vi "NISE.Reserve.vi"(0 "SLSC Interface in":refnum<class "SLSC Interface.lvclass">, 5 "devices":refnum<k21>="$DefaultDevices", 7 "reservation access (Read/Write)":i32(ring)=3 items=["Read Only"=1, "Read/Write"=3], 9 "reservation group":string, 11 "error in (no error)":errorcluster) -> (4 "SLSC Interface out":refnum<class "SLSC Interface.lvclass">, 15 "error out":errorcluster)   [LabVIEW 2016, in "SLSC Interface.lvclass"]
uses:
  SLSC Interface.lvclass
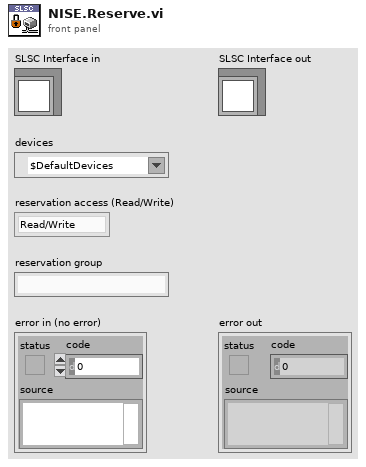
[diagram p1: front panel]
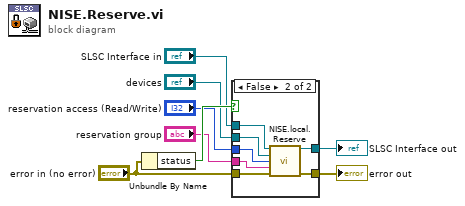
[diagram p0: block diagram]
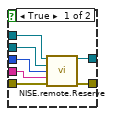
[diagram p2: hidden frame]
diagram:
  n1 = Unbundle By Name("error in (no error)") -> ("status"=w8:bool)
  n2 = case shown="False" w8 {
    tunnel: "SLSC Interface in" -> [w15 w22]
    tunnel: [w14 w21] -> w6
    tunnel: "devices" -> [w13 w20]
    tunnel: "reservation access (Read/Write)" -> [w12 w19]
    tunnel: "reservation group" -> [w11 w18]
    tunnel: "error in (no error)" -> [w10 w17]
    tunnel: [w9 w16] -> w1
    frame True {
      n3 = call "NISE.remote.Reserve.vi"("SLSC Remote in"=w15, "devices"=w13, "reservation access (Read/Write)"=w12, "reservation group"=w11, "error in (no error)"=w10) -> ("SLSC Remote out"=w14:refnum<class "SLSC Interface.lvclass">, "error out"=w9:errorcluster)  [unwired: 9 in]
    }
    frame False {
      n4 = call "NISE.local.Reserve.vi"("SLSC Local in"=w22, "devices"=w20, "reservation access (Read/Write)"=w19, "reservation group"=w18, "error in (no error)"=w17) -> ("SLSC Local out"=w21:refnum<class "SLSC Interface.lvclass">, "error out"=w16:errorcluster)  [unwired: 9 in]
    }
  }
  "error out" <- w1
  "SLSC Interface out" <- w6
